vi "Get Document Path.vi"(8 "error in (no error)":errorcluster, 11 "Document API in":refnum<class "Document API.lvclass">) -> (0 "error out":errorcluster, 2 "Document Path":path, 3 "Document API out":refnum<class "Document API.lvclass">)   [LabVIEW 2017, in "Document API.lvlib" / "Document API.lvclass"]
doc: "i"
uses:
  Document API.lvclass
  Document API.lvclass/Document API.ctl
  NPOI_Document/npoiDocument/npoiDocument.lvclass/npoiDocument.ctl
  NPOI_Document/npoiDocument/Get Document.Path.vi
  NPOI_Document/npoiDocument/npoiDocument.lvclass
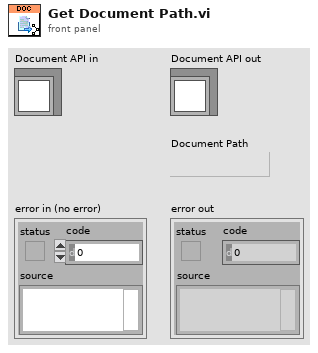
[diagram p1: front panel]
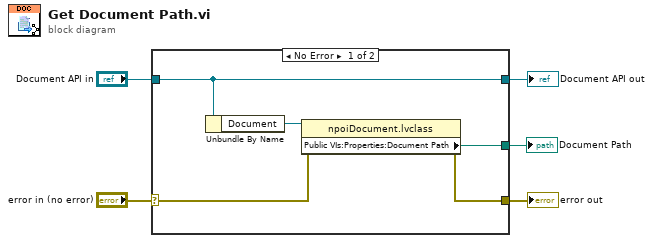
[diagram p0: block diagram]
diagram:
  n1 = case shown="No Error" "error in (no error)" {
    selector: "error in (no error)" -> [w7 w12]
    tunnel: [w6 w12] -> w4
    tunnel: [w10 w11] -> w2
    tunnel: "Document API in" -> [w10 w11]
    tunnel: [w8 _] -> w1
    frame No Error {
      n2 = Unbundle By Name(w10) -> ("Document"=w9:refnum<class "npoiDocument.lvclass">)
      n3 = property class="npoiDocument.lvclass"(reference=w9, error in=w7) -> (error out=w6:errorcluster, "Public VIs:Properties:Document Path"=w8:path)  [unwired: 1 out]
    }
    frame Error {
    }
  }
  "error out" <- w4
  "Document API out" <- w2
  "Document Path" <- w1
